vi "Update Msj.vi"(8 "error in (no error)":errorcluster, 10 "Update Msj":string, 11 "Mensajes Actor in":refnum<class "Mensajes Actor.lvclass">) -> (0 "error out":errorcluster, 3 "Mensajes Actor out":refnum<class "Mensajes Actor.lvclass">)   [LabVIEW 2019, in "Mensajes Actor.lvlib" / "Mensajes Actor.lvclass"]
uses:
  Mensajes Actor.lvclass
  Mensajes Actor.lvclass/Mensajes Actor.ctl
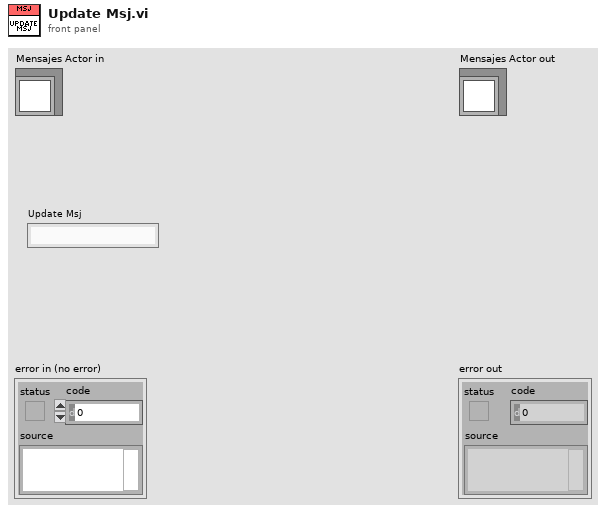
[diagram p1: front panel]
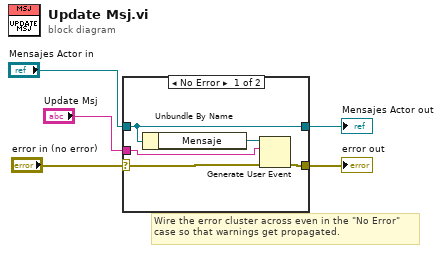
[diagram p0: block diagram]
diagram:
  # "Wire the error cluster across even in the \"No Error\"\ncase so that warnings get propagated."
  n1 = case shown="No Error" "error in (no error)" {
    selector: "error in (no error)" -> [w8 w12]
    tunnel: [w7 w12] -> w4
    tunnel: [w10 w11] -> w2
    tunnel: "Mensajes Actor in" -> [w10 w11]
    tunnel: "Update Msj" -> [w6 _]
    frame No Error {
      n2 = Unbundle By Name(w10) -> ("Mensaje"=w9:refnum<user-event>)
      n3 = Generate User Event(user event=w9, event data cluster=w6, error in=w8) -> (error out=w7:errorcluster)  [unwired: 1 in, 1 out]
    }
    frame Error {
    }
  }
  "error out" <- w4
  "Mensajes Actor out" <- w2
